vi "save_log_file.vi"(11 "msg":refnum<vi>) -> ()   [LabVIEW 2016, in "MotionControl_UFO_3DOF.lvlib"]
uses:
  <userlib>/MotionControl_UFO_3DOF/MotionControl_UFO_3DOF.lvlib
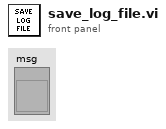
[diagram p1: front panel]
types:
  T1 = enum16{"open", "replace", "create", "open or create", "replace or create", "replace or create with confirmation"}
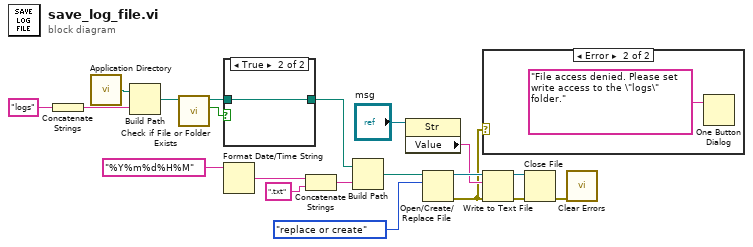
[diagram p0: block diagram]
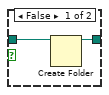
[diagram p3: hidden frame]
diagram:
  n1 = Concatenate Strings("logs") -> (w14:string)
  n2 = call <vilib>:"Application Directory.vi"() -> ("Application Directory"=w9:path)
  n3 = Build Path(base path=w9, name or relative path=w14) -> (appended path=w17:path)
  n4 = call <vilib>:"Check if File or Folder Exists.vi"("path"=w17) -> ("file or folder exists?"=w18:bool, "dup path"=w19:path)  [unwired: 8 in, 1 out]
  n5 = case shown="True" w18 {
    tunnel: w19 -> [w22 w23]
    tunnel: [w21 w23] -> w20
    frame False {
      n6 = Create Folder(path (use dialog)=w22) -> (created path=w21:path)  [unwired: 2 in, 2 out]
    }
    frame True {
    }
  }
  n7 = Format Date/Time String(time format string (%c)="%Y%m%d%H%M" ("时间格式字符串(%c)")) -> (date/time string=w6:string)  [unwired: 2 in]
  n8 = Concatenate Strings(w6, ".txt") -> (w5:string)
  n9 = Build Path(base path=w20, name or relative path=w5) -> (appended path=w8:path)
  n10 = property on="属性节点" class="Str"(reference="msg") -> ("Value"=w11:string)  [unwired: 1 in, 2 out]
  n11 = Open/Create/Replace File(file path (use dialog)=w8, operation (0:open)=T1."replace or create" ("操作(0:open)")) -> (refnum out=w12:refnum<file>, error out=w2:errorcluster)  [unwired: 4 in, 1 out]
  n12 = case shown="Error" w2 {
    frame No Error {
    }
    frame Error {
      n13 = One Button Dialog(message="File access denied. Please set write access to the \"logs\" folder.") -> ()  [unwired: 1 in, 1 out]
    }
  }
  n14 = Write to Text File(file (use dialog)=w12, text=w11, error in=w2) -> (refnum out=w10:refnum<file>, error out=w3:errorcluster)  [unwired: 1 in, 1 out]
  n15 = Close File(refnum=w10, error in=w3) -> (error out=w1:errorcluster)  [unwired: 1 out]
  n16 = call <vilib>:"Clear Errors.vi"("error in (no error)"=w1) -> ()  [unwired: 5 in, 2 out]
